vi "RefreshRecipeUI.vi"(7 "TorqueUnit":string, 8 "PIDAdj":refnum<vi>, 9 "MultiPointFunc":refnum<vi>, 10 "LoadWaveform":refnum<vi>, 11 "refTestPara":refnum<vi>) -> ()   [LabVIEW 2016]
uses:
  MFActor/TestParameter.ctl
panel:
  in  "TestPara":T1={"LoadType"=enum."15kW Servo Motor", "TestItem"=0, "Program_Multi"=0, "Crest"=0.0, "TestSpeed"=0.0, "Trugh"=0.0, "PID"={"NP"=0.0, "NI"=0.0, "ND"=0.0, "NPS"="A", "NIS"="A", "NDS"="A"}, "LoadValue"=0.0, "Period"=0.0, "DataFetchRate"=0.0, "TestPtData"=[]} {"DataFetchRate" format="%#_2f"; "Period" format="%#_2f"; "LoadValue" format="%#_2f"; "PID"."ND" min=0.0 max=99.0 format="%#.2f"; "PID"."NI" min=0.0 max=99.0 step=1.0 format="%#.2f"; "PID"."NP" min=0.0 max=99.0 format="%#.2f"; "Trugh" format="%#_2f"; "TestSpeed" format="%#_2f"; "Crest" format="%#_2f"}
  out "PID":refnum<vi>
  out "DataFetchRate":refnum<vi>
  out "LoadValue":refnum<vi>
  out "Period":refnum<vi>
  out "Trugh":refnum<vi>
  out "Crest":refnum<vi>
  out "TestSpeed":refnum<vi>
  out "Program_Multi":refnum<vi>
  out "TestItem":refnum<vi>
  out "LoadType":refnum<vi>
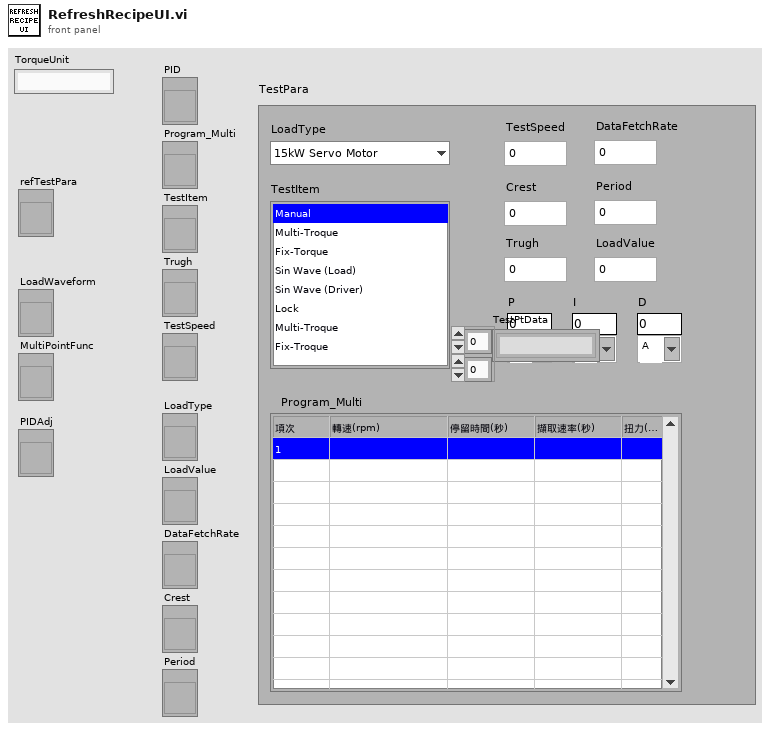
[diagram p1: front panel]
types:
  T1 = typedef "TestParameter.ctl" = cluster{"LoadType":enum16{"15kW Servo Motor", "Brake"}, "TestItem":i32, "Program_Multi":i32, "Crest":dbl, "TestSpeed":dbl, "Trugh":dbl, "PID":cluster{"NP":dbl, "NI":dbl, "ND":dbl, "NPS":string, "NIS":string, "NDS":string}, "LoadValue":dbl, "Period":dbl, "DataFetchRate":dbl, "TestPtData":string[][]}
  T2 = enum8{"Enabled", "Disabled", "Disabled and Grayed Out"}
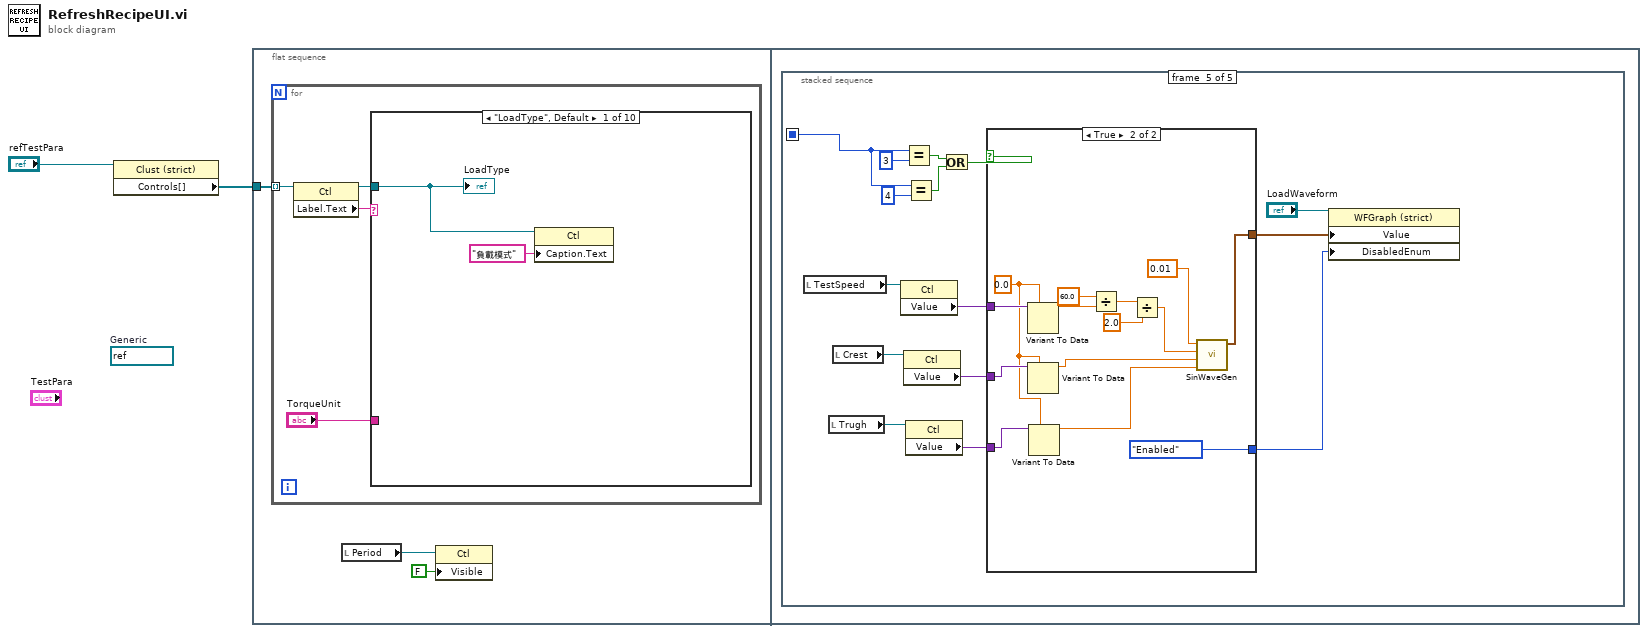
[diagram p0: block diagram]
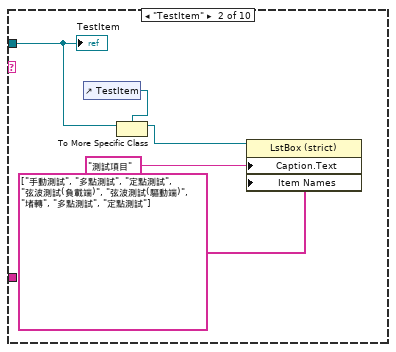
[diagram p2: hidden frame]
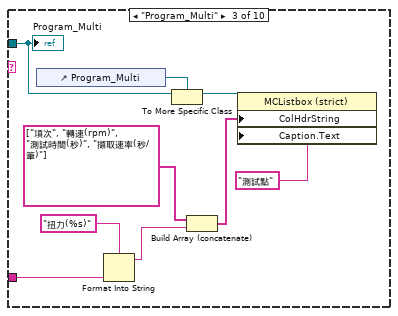
[diagram p3: hidden frame]
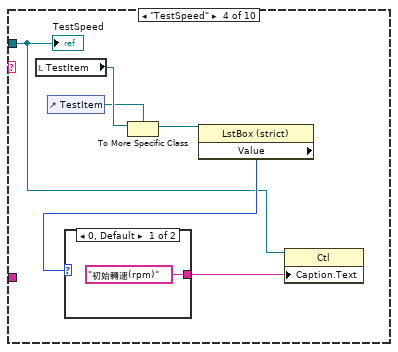
[diagram p4: hidden frame]
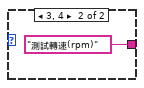
[diagram p5: hidden frame]
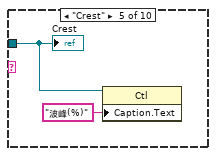
[diagram p6: hidden frame]
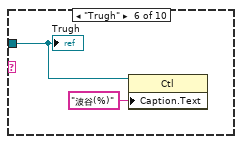
[diagram p7: hidden frame]
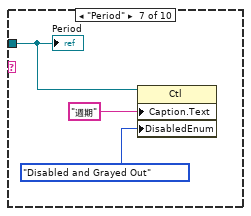
[diagram p8: hidden frame]
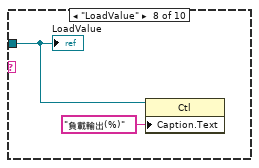
[diagram p9: hidden frame]
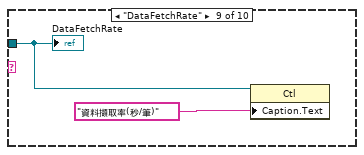
[diagram p10: hidden frame]
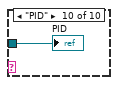
[diagram p11: hidden frame]
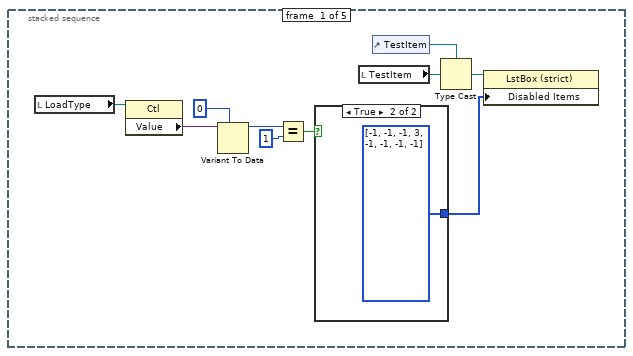
[diagram p12: hidden frame]
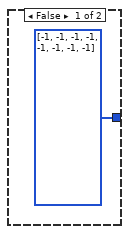
[diagram p13: hidden frame]
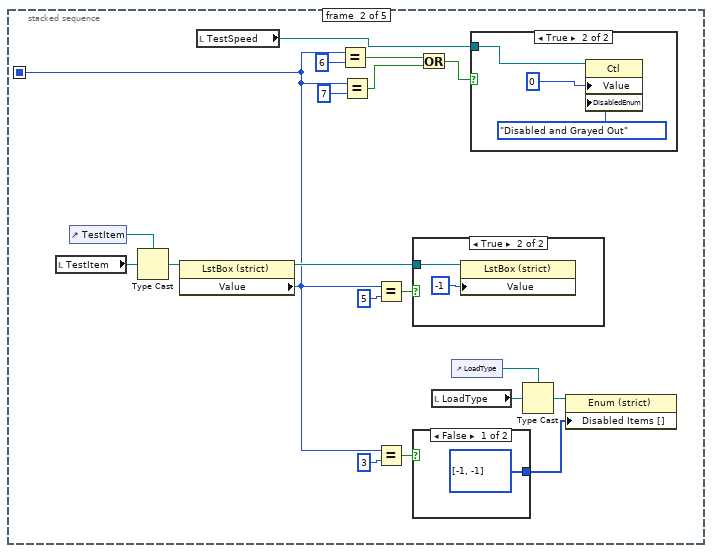
[diagram p14: hidden frame]
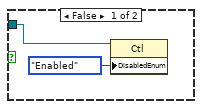
[diagram p15: hidden frame]
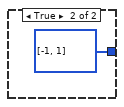
[diagram p16: hidden frame]
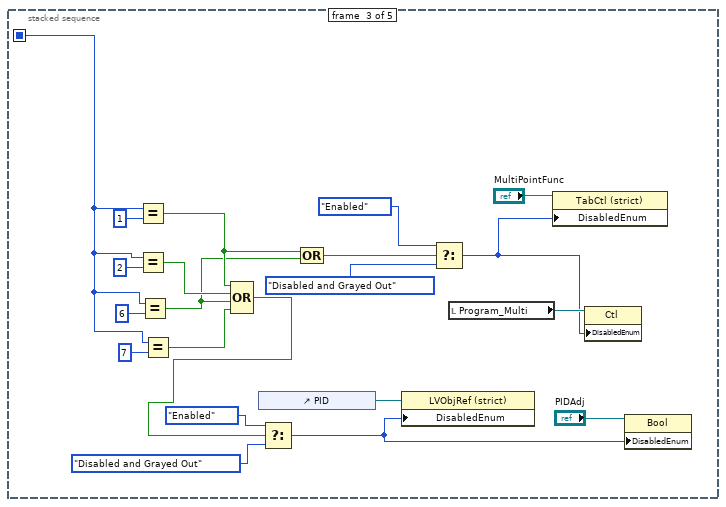
[diagram p18: hidden frame]
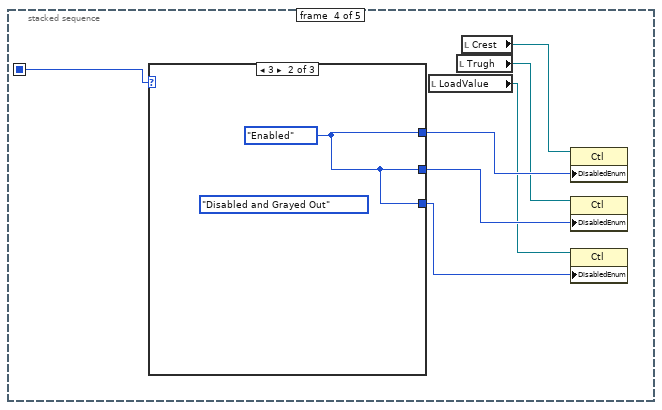
[diagram p19: hidden frame]
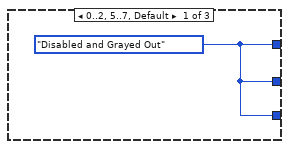
[diagram p20: hidden frame]
diagram:
  (unwired) refnum<vi> refnum  # Generic
  n1 = property class="Clust (strict)"(reference="refTestPara") -> ("Controls[]"=w2:refnum<vi>[])  [unwired: 1 in, 2 out]
  n2 = flat-sequence {
    tunnel: w2 -> [w5]
    frame #0 {
      n3 = for {
        tunnel: w5 -> [w9] mode=indexing
        n4 = property class="Ctl"(reference=w9) -> (reference out=w7:refnum<vi>, "Label.Text"=w8:string)  [unwired: 1 in, 1 out]
        n5 = case shown="\"LoadType\", Default" w8 {
          tunnel: w7 -> [w11 w15 w25 w27 w35 w36 w39 w41 w44 w45]
          tunnel: "TorqueUnit" -> [_ _ w20 _ _ _ _ _ _ _]
          frame "LoadType", Default {
            n6 = property class="Ctl"(reference=w11, "Caption.Text"="負載模式") -> ()  [unwired: 1 in, 2 out]
            "LoadType" <- w11
          }
          frame "TestItem" {
            n7 = control-ref of="TestItem"() -> (w16:refnum<vi>)
            n8 = To More Specific Class(target class=w16, reference=w15) -> (specific class reference=w14:refnum<vi>)  [unwired: 1 in, 1 out]
            n9 = property class="LstBox (strict)"(reference=w14, "Caption.Text"="測試項目", "Item Names"=string[] ["手動測試", "多點測試", "定點測試", "弦波測試(負載端)", "弦波測試(驅動端)", "堵轉", "多點測試", "定點測試"]) -> ()  [unwired: 1 in, 2 out]
            "TestItem" <- w15
          }
          frame "Program_Multi" {
            n10 = control-ref of="Program_Multi"() -> (w24:refnum<vi>)
            n11 = Format Into String(format string="扭力(%s)", w20) -> (resulting string=w19:string)  [unwired: 2 in, 1 out]
            n12 = To More Specific Class(target class=w24, reference=w25) -> (specific class reference=w23:refnum<vi>)  [unwired: 1 in, 1 out]
            n13 = Build Array (concatenate)(string[] ["項次", "轉速(rpm)", "測試時間(秒)", "擷取速率(秒/筆)"] ("Column Header Strings[]"), w19) -> (w18:string[])
            n14 = property class="MCListbox (strict)"(reference=w23, "ColHdrString"=w18, "Caption.Text"="測試點") -> ()  [unwired: 1 in, 2 out]
            "Program_Multi" <- w25
          }
          frame "TestSpeed" {
            n15 = local read "TestItem"() -> (w31:refnum<vi>)
            n16 = control-ref of="TestItem"() -> (w30:refnum<vi>)
            n17 = To More Specific Class(target class=w30, reference=w31) -> (specific class reference=w29:refnum<vi>)  [unwired: 1 in, 1 out]
            n18 = property class="LstBox (strict)"(reference=w29) -> ("Value"=w28:i32)  [unwired: 1 in, 2 out]
            n19 = case shown="0, Default" w28 {
              tunnel: ["初始轉速(rpm)" "測試轉速(rpm)"] -> w26
              frame 0, Default {
              }
              frame 3, 4 {
              }
            }
            n20 = property class="Ctl"(reference=w27, "Caption.Text"=w26) -> ()  [unwired: 1 in, 2 out]
            "TestSpeed" <- w27
          }
          frame "Crest" {
            n21 = property class="Ctl"(reference=w35, "Caption.Text"="波峰(%)") -> ()  [unwired: 1 in, 2 out]
            "Crest" <- w35
          }
          frame "Trugh" {
            n22 = property class="Ctl"(reference=w36, "Caption.Text"="波谷(%)") -> ()  [unwired: 1 in, 2 out]
            "Trugh" <- w36
          }
          frame "Period" {
            n23 = property class="Ctl"(reference=w39, "Caption.Text"="週期", "DisabledEnum"=T2."Disabled and Grayed Out" ("Disabled")) -> ()  [unwired: 1 in, 2 out]
            "Period" <- w39
          }
          frame "LoadValue" {
            n24 = property class="Ctl"(reference=w41, "Caption.Text"="負載輸出(%)") -> ()  [unwired: 1 in, 2 out]
            "LoadValue" <- w41
          }
          frame "DataFetchRate" {
            n25 = property class="Ctl"(reference=w44, "Caption.Text"="資料擷取率(秒/筆)") -> ()  [unwired: 1 in, 2 out]
            "DataFetchRate" <- w44
          }
          frame "PID" {
            "PID" <- w45
          }
        }
      }
      n26 = local read "Period"() -> (w4:refnum<vi>)
      n27 = property class="Ctl"(reference=w4, "Visible"=FALSE) -> ()  [unwired: 1 in, 2 out]
    }
    frame #1 {
      n28 = stacked-sequence {
        seq-local: [_ w64 _ _ _] -> [_ _ w86 w113 w131]
        frame #0 {
          n29 = local read "LoadType"() -> (w55:refnum<vi>)
          n30 = property class="Ctl"(reference=w55) -> ("Value"=w54:variant)  [unwired: 1 in, 2 out]
          n31 = Variant To Data(type=u16 0, Variant=w54) -> (data=w52:u16)  [unwired: 1 in, 1 out]
          n32 = Equal?(x=w52, y=u16 1) -> (x = y?=w50:bool)
          n33 = case shown="True" w50 {
            tunnel: [i32[] [-1, -1, -1, -1, -1, -1, -1, -1] ("Disabled Items") i32[] [-1, -1, -1, 3, -1, -1, -1, -1] ("Disabled Items")] -> w46
            frame False {
            }
            frame True {
            }
          }
          n34 = local read "TestItem"() -> (w47:refnum<vi>)
          n35 = control-ref of="TestItem"() -> (w48:refnum<vi>)
          n36 = Type Cast(type=w48, x=w47) -> (*(type *) &x=w49:refnum<vi>)
          n37 = property class="LstBox (strict)"(reference=w49, "Disabled Items"=w46) -> ()  [unwired: 1 in, 2 out]
        }
        frame #1 {
          n38 = local read "TestItem"() -> (w74:refnum<vi>)
          n39 = control-ref of="TestItem"() -> (w75:refnum<vi>)
          n40 = Type Cast(type=w75, x=w74) -> (*(type *) &x=w76:refnum<vi>)
          n41 = property class="LstBox (strict)"(reference=w76) -> (reference out=w65:refnum<vi>, "Value"=w64:i32)  [unwired: 1 in, 1 out]
          n42 = local read "TestSpeed"() -> (w59:refnum<vi>)
          n43 = Equal?(x=w64, y=6) -> (x = y?=w61:bool)
          n44 = Equal?(x=w64, y=7) -> (x = y?=w60:bool)
          n45 = Equal?(x=w64, y=5) -> (x = y?=w71:bool)
          n46 = Equal?(x=w64, y=3) -> (x = y?=w70:bool)
          n47 = case shown="True" w71 {
            tunnel: w65 -> [_ w85]
            frame False {
            }
            frame True {
              n48 = property class="LstBox (strict)"(reference=w85, "Value"=-1) -> ()  [unwired: 1 in, 2 out]
            }
          }
          n49 = case shown="False" w70 {
            tunnel: [i32[] [-1, -1] ("Disabled Items []") i32[] [-1, 1] ("Disabled Items []")] -> w66
            frame False {
            }
            frame True {
            }
          }
          n50 = Or(x=w61, y=w60) -> (x .or. y?=w58:bool)
          n51 = local read "LoadType"() -> (w69:refnum<vi>)
          n52 = control-ref of="LoadType"() -> (w68:refnum<vi>)
          n53 = case shown="True" w58 {
            tunnel: w59 -> [w78 w81]
            frame False {
              n54 = property class="Ctl"(reference=w78, "DisabledEnum"=T2."Enabled" ("Disabled")) -> ()  [unwired: 1 in, 2 out]
            }
            frame True {
              n55 = property class="Ctl"(reference=w81, "Value"=0, "DisabledEnum"=T2."Disabled and Grayed Out" ("Disabled")) -> ()  [unwired: 1 in, 2 out]
            }
          }
          n56 = Type Cast(type=w68, x=w69) -> (*(type *) &x=w67:refnum<vi>)
          n57 = property class="Enum (strict)"(reference=w67, "Disabled Items []"=w66) -> ()  [unwired: 1 in, 2 out]
        }
        frame #2 {
          n58 = Equal?(x=w86, y=1) -> (x = y?=w96:bool)
          n59 = Equal?(x=w86, y=2) -> (x = y?=w102:bool)
          n60 = Equal?(x=w86, y=6) -> (x = y?=w95:bool)
          n61 = Equal?(x=w86, y=7) -> (x = y?=w101:bool)
          n62 = Compound Arithmetic op=OR(w96, w102, w95, w101) -> (w97:bool)
          n63 = control-ref of="PID"() -> (w100:refnum<vi>)
          n64 = Select(t=T2."Enabled" ("Disabled"), s=w97, f=T2."Disabled and Grayed Out" ("Disabled")) -> (s? t:f=w89:T2)
          n65 = Compound Arithmetic op=OR(w96, w95) -> (w93:bool)
          n66 = property class="LVObjRef (strict)"(reference=w100, "DisabledEnum"=w89) -> ()  [unwired: 1 in, 2 out]
          n67 = Select(t=T2."Enabled" ("Disabled"), s=w93, f=T2."Disabled and Grayed Out" ("Disabled")) -> (s? t:f=w87:T2)
          n68 = local read "Program_Multi"() -> (w94:refnum<vi>)
          n69 = property class="TabCtl (strict)"(reference="MultiPointFunc", "DisabledEnum"=w87) -> ()  [unwired: 1 in, 2 out]
          n70 = property class="Ctl"(reference=w94, "DisabledEnum"=w87) -> ()  [unwired: 1 in, 2 out]
          n71 = property class="Bool"(reference="PIDAdj", "DisabledEnum"=w89) -> ()  [unwired: 1 in, 2 out]
        }
        frame #3 {
          n72 = case shown="3" w113 {
            tunnel: [w114 w115 w116] -> w112
            tunnel: [w114 w115 w116] -> w111
            tunnel: [w114 w115 w116] -> w110
            frame 0..2, 5..7, Default {
              w114 = T2."Disabled and Grayed Out" ("Disabled")
            }
            frame 3 {
              (unwired) T2."Disabled and Grayed Out" ("Disabled")
              w115 = T2."Enabled" ("Disabled")
            }
            frame 4 {
              w116 = T2."Enabled" ("Disabled")
            }
          }
          n73 = local read "LoadValue"() -> (w109:refnum<vi>)
          n74 = local read "Trugh"() -> (w108:refnum<vi>)
          n75 = local read "Crest"() -> (w107:refnum<vi>)
          n76 = property class="Ctl"(reference=w107, "DisabledEnum"=w112) -> ()  [unwired: 1 in, 2 out]
          n77 = property class="Ctl"(reference=w108, "DisabledEnum"=w111) -> ()  [unwired: 1 in, 2 out]
          n78 = property class="Ctl"(reference=w109, "DisabledEnum"=w110) -> ()  [unwired: 1 in, 2 out]
        }
        frame #4 {
          n79 = local read "TestSpeed"() -> (w124:refnum<vi>)
          n80 = local read "Trugh"() -> (w117:refnum<vi>)
          n81 = local read "Crest"() -> (w123:refnum<vi>)
          n82 = property class="Ctl"(reference=w124) -> ("Value"=w122:variant)  [unwired: 1 in, 2 out]
          n83 = Equal?(x=w131, y=3) -> (x = y?=w128:bool)
          n84 = property class="Ctl"(reference=w123) -> ("Value"=w121:variant)  [unwired: 1 in, 2 out]
          n85 = Equal?(x=w131, y=4) -> (x = y?=w127:bool)
          n86 = property class="Ctl"(reference=w117) -> ("Value"=w120:variant)  [unwired: 1 in, 2 out]
          n87 = Or(x=w128, y=w127) -> (x .or. y?=w125:bool)
          n88 = case shown="True" w125 {
            tunnel: w122 -> [_ w142]
            tunnel: w121 -> [_ w141]
            tunnel: w120 -> [_ w140]
            tunnel: [_ w134] -> w119
            tunnel: [T2."Disabled and Grayed Out" ("Disabled") T2."Enabled" ("Disabled")] -> w118
            frame False {
            }
            frame True {
              w139 = 0.0
              n89 = Variant To Data(type=w139, Variant=w142) -> (data=w143:dbl)  [unwired: 1 in, 1 out]
              n90 = Variant To Data(type=w139, Variant=w141) -> (data=w136:dbl)  [unwired: 1 in, 1 out]
              n91 = Variant To Data(type=w139, Variant=w140) -> (data=w135:dbl)  [unwired: 1 in, 1 out]
              n92 = Divide(x=60.0, y=w143) -> (x/y=w145:dbl)
              n93 = Divide(x=w145, y=2.0) -> (x/y=w137:dbl)
              n94 = call "SinWaveGen.vi"("WaveTrough"=w135, "WaveCrest"=w136, "SinWavePeriod(Sec)"=w137, "dt"=0.01) -> ("Waveform"=w134:waveform(dbl))  [unwired: 6 in, 1 out]
            }
          }
          n95 = property class="WFGraph (strict)"(reference="LoadWaveform", "Value"=w119, "DisabledEnum"=w118) -> ()  [unwired: 1 in, 2 out]
        }
      }
    }
  }
